vi "New Error Pointer.vi"(8 "error in (no error)":errorcluster, 11 "count (1)":u64=1) -> (0 "error out":errorcluster, 3 "Error Pointer":refnum<class "Error Pointer.lvclass">)   [LabVIEW 2019, in "DSF Core.lvlib" / "Error Pointer.lvclass"]
uses:
  Error Pointer.lvclass
  C:/Program Files (x86)/National Instruments/LabVIEW 2019/vi.lib/NI/Memory Manager/Classes/Pointer/Pointer.lvclass
  Error Sizes.ctl
  <vilib>/NI/Memory Manager/Classes/Pointer/Pointer.lvclass/Pointer.ctl
  Error Pointer.lvclass/Error Pointer.ctl
  <vilib>/NI/Memory Manager/Classes/Pointer/Set Address.vi
  <vilib>/NI/Memory Manager/Classes/Pointer/Set Size.vi
  <vilib>/NI/Memory Manager/Classes/Pointer/Set Internal.vi
  <vilib>/NI/Memory Manager/Classes/Pointer/Write.vi
  <vilib>/NI/Memory Manager/Classes/Pointer/Write 1D U8.vi
  <vilib>/NI/Memory Manager/Classes/Pointer/Clear.vi
  Get Power Of 2.vi
  <vilib>/NI/Memory Manager/Classes/Pointer/Write (No Check).vi
  <vilib>/NI/Memory Manager/Classes/Pointer/Write (No Check) 1D U8.vi
  <vilib>/NI/Memory Manager/Classes/Pointer/Check Move.vi
  <vilib>/NI/Memory Manager/Classes/Pointer/Check Null Pointer.vi
  <vilib>/NI/Memory Manager/Classes/Pointer/Clear (No Check).vi
  <vilib>/NI/Memory Manager/Classes/Pointer/Check Length.vi
  <vilib>/NI/Memory Manager/Classes/Pointer/Get Address.vi
  <vilib>/NI/Memory Manager/Classes/Pointer/Check Count.vi
  <vilib>/NI/Memory Manager/Classes/Pointer/Check Bounds (Power of 2).vi
  <vilib>/NI/Memory Manager/Classes/Pointer/Errors.vi
  <vilib>/NI/Memory Manager/Classes/Pointer/Null Pointer.vi
  <vilib>/NI/Memory Manager/Classes/Pointer/Is Null.vi
  <vilib>/NI/Memory Manager/Classes/Pointer/Get Size.vi
  <vilib>/NI/Memory Manager/Classes/Pointer/Check Bounds (Pointer).vi
  <vilib>/NI/Memory Manager/Classes/Pointer/Out of Bounds.vi
  <vilib>/NI/Memory Manager/Classes/Pointer/Check Bounds.vi
  <vilib>/NI/Memory Manager/Classes/Pointer/Create Error.vi
  <vilib>/NI/Memory Manager/VIs/Write String to Source.vi
  <vilib>/NI/Memory Manager/Classes/Pointer/Write Pointer Size to Error.vi
  <vilib>/NI/Memory Manager/VIs/Write Numeric to Source.vi
  <vilib>/NI/Memory Manager/VIs/Write Numeric Scalar to Source (Base10 U64).vi
  <vilib>/NI/Memory Manager/Classes/Pointer/Check Bounds (Buffer).vi
  <vilib>/NI/Memory Manager/VIs/New Error Cluster.vi
  <vilib>/NI/Memory Manager/VIs/New Error Cluster (512B).vi
  <vilib>/NI/Memory Manager/VIs/Set Error Status.vi
  <vilib>/NI/Memory Manager/VIs/Set Error Code.vi
  <vilib>/NI/Memory Manager/VIs/Set Error Source.vi
  <vilib>/NI/Memory Manager/Constants/Constants.vi
  <vilib>/NI/Memory Manager/Constants/Library Name.vi
  <vilib>/NI/Memory Manager/Classes/Pointer/Pointer Error Info.vi
  <vilib>/NI/Memory Manager/Constants/Pointer Class Name.vi
  <vilib>/NI/Memory Manager/Classes/Pointer/Buffer Underflow.vi
  <vilib>/NI/Memory Manager/Classes/Pointer/Pointer.lvclass
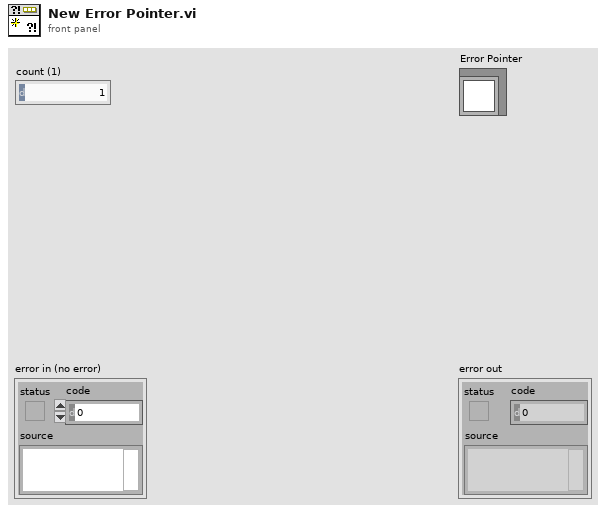
[diagram p1: front panel]
types:
  T1 = typedef "DSF Core.lvlib/Error Pointer.lvclass/Error Sizes.ctl" = enum8{"256", "512", "1024"}
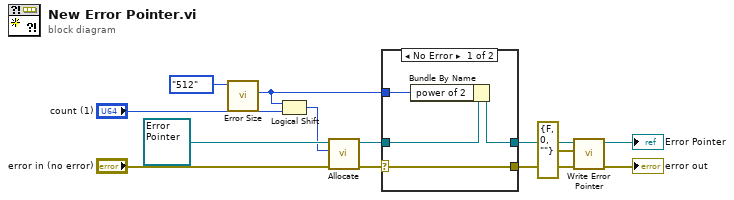
[diagram p0: block diagram]
diagram:
  n1 = call "Error Size.vi"("error size"=Error_Sizes."512") -> ("power of 2"=w2:i16)  [unwired: 9 in, 1 out]
  n2 = Logical Shift(y=w2, x="count (1)") -> (x << y=w1:u64)
  n3 = call <vilib>:"Allocate.vi"("error in (no error)"="error in (no error)", "size"=w1, "Pointer type"=refnum<class "Error Pointer.lvclass"> refnum ("Error Pointer in")) -> ("error out"=w8:errorcluster, "Pointer out"=w7:refnum<class "Error Pointer.lvclass">)  [unwired: 7 in]
  n4 = case shown="No Error" w8 {
    selector: w8 -> [w14 w18]
    tunnel: w7 -> [w17 w19]
    tunnel: w2 -> [w16 _]
    tunnel: [w15 w19] -> w5
    tunnel: [w14 w18] -> w4
    frame No Error {
      n5 = Bundle By Name(cluster=w17, "power of 2"=w16) -> (w15:refnum<class "Error Pointer.lvclass">)
    }
    frame Error {
    }
  }
  n6 = call "Write Error Pointer.vi"("error in (no error)"=w4, "error"=errorcluster {"status"=FALSE, "code"=0, "source"=""}, "Error Pointer in"=w5) -> ("error out"=→"error out":errorcluster, "Error Pointer in"=→"Error Pointer":refnum<class "Error Pointer.lvclass">)  [unwired: 7 in]
